vi "Move Labels in Menu.vi"(8 "error in (no error)":errorcluster caption="错误输入（无错误）", 10 "标签位置":i32[](array[numeric]), 11 "图形对象":refnum<vi>[](array[refnum])) -> (0 "error out":errorcluster caption="错误输出")   [LabVIEW 2020]
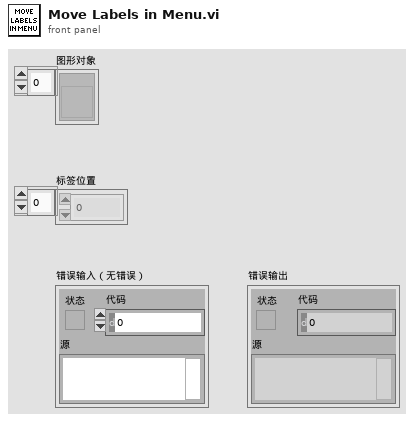
[diagram p1: front panel]
types:
  T1 = typedef "LVRectTypeDef.ctl" = cluster{"Left":i16, "Top":i16, "Right":i16, "Bottom":i16}
  T2 = cluster{"MasterRect":T1, "Label":refnum<vi>, "s? t:f":i32, refnum<vi>}
  T3 = enum32{"None", "Size to Fit", "Arrange Horizontally", "Arrange Vertically"}
  T4 = cluster{"Bounds Rect":T1, "Label":refnum<vi>, "s? t:f":i32, refnum<vi>}
  T5 = cluster{"Bounds Rect":T1, "Label":refnum<vi>, "right-top":i32, refnum<vi>}
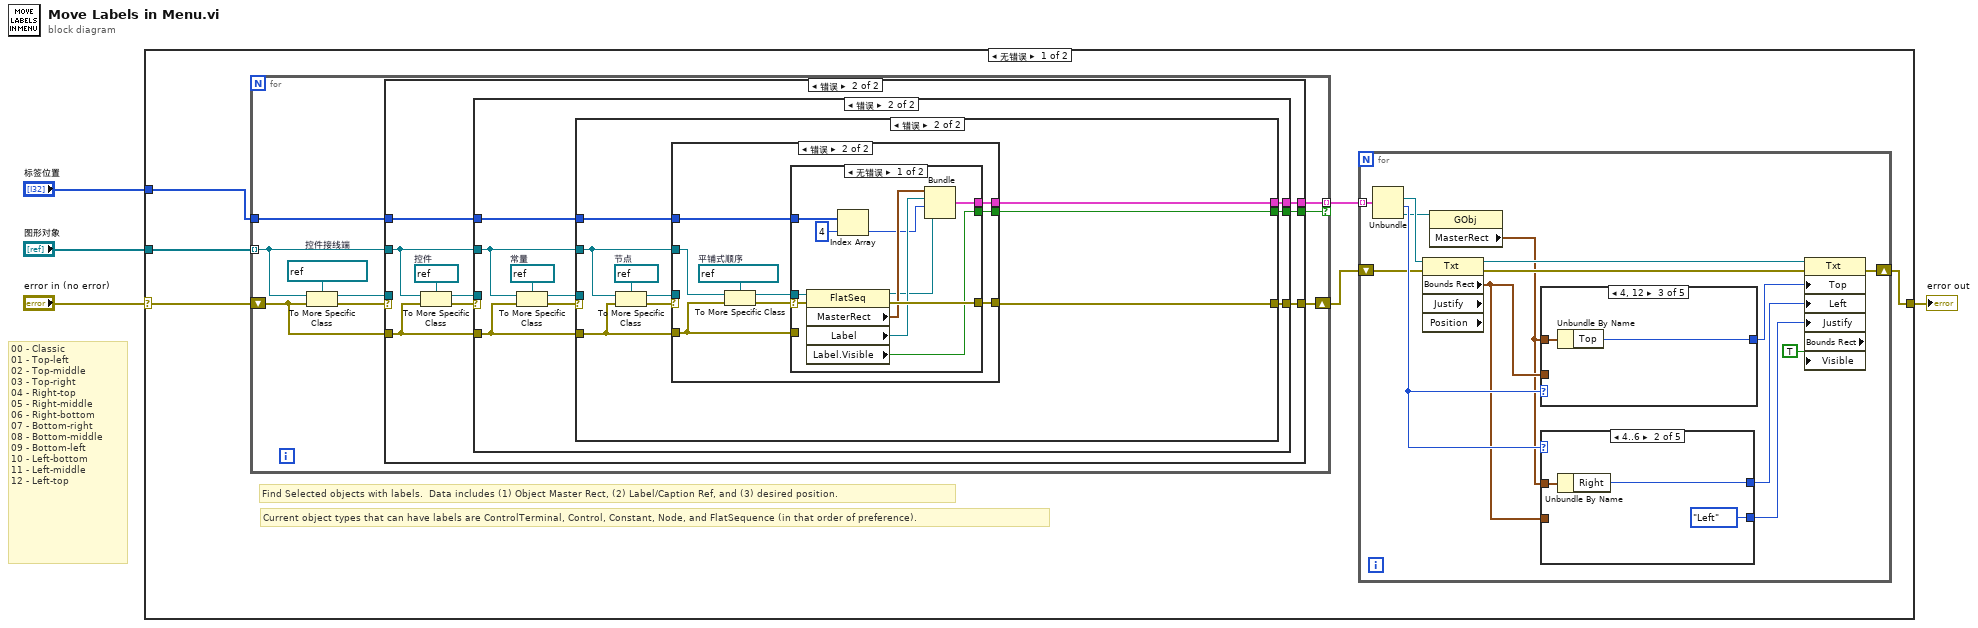
[diagram p0: block diagram]
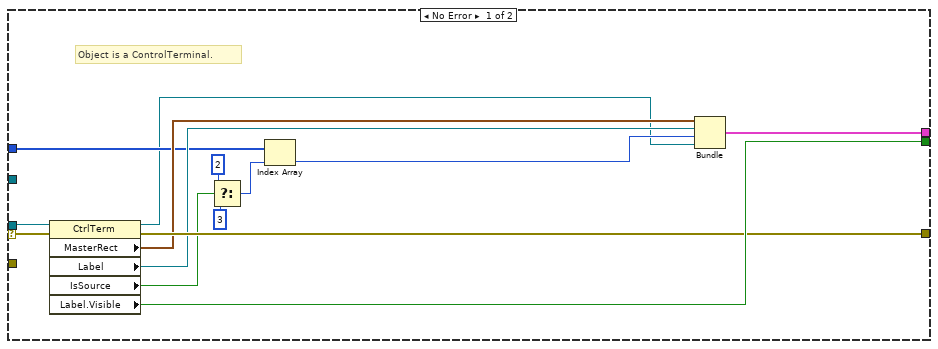
[diagram p2: hidden frame]
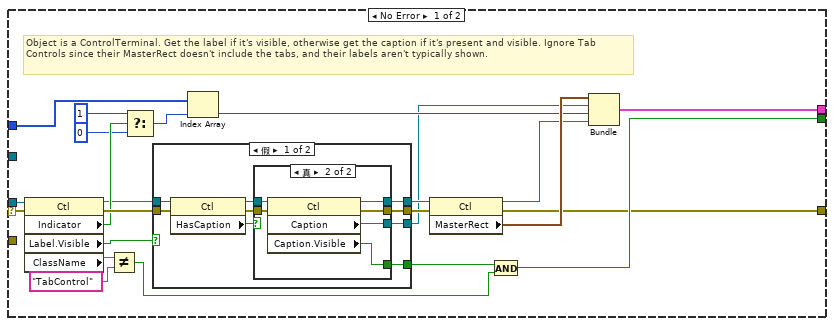
[diagram p3: hidden frame]
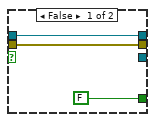
[diagram p4: hidden frame]
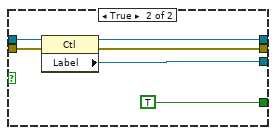
[diagram p5: hidden frame]
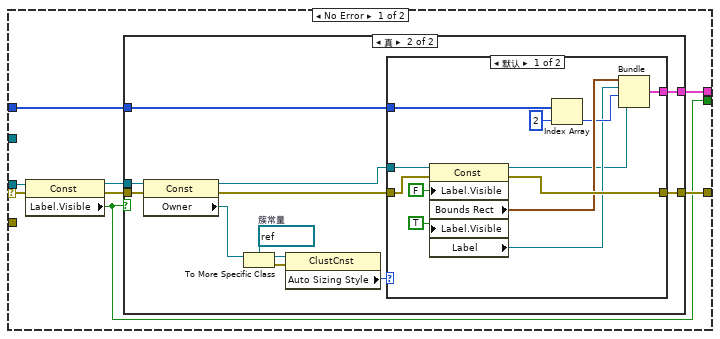
[diagram p6: hidden frame]
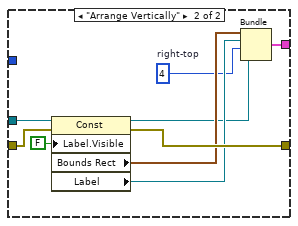
[diagram p8: hidden frame]
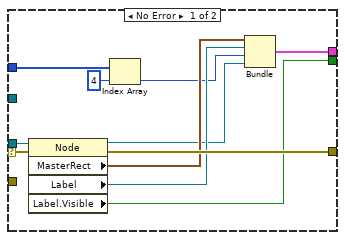
[diagram p9: hidden frame]
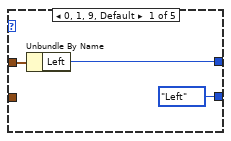
[diagram p11: hidden frame]
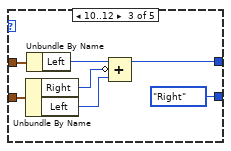
[diagram p12: hidden frame]
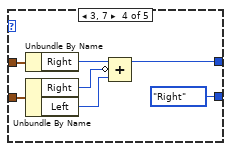
[diagram p13: hidden frame]
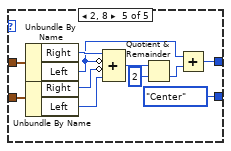
[diagram p14: hidden frame]
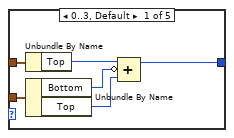
[diagram p15: hidden frame]
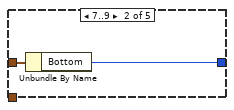
[diagram p16: hidden frame]
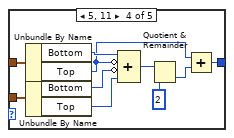
[diagram p17: hidden frame]
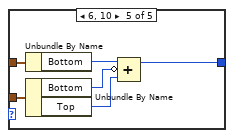
[diagram p18: hidden frame]
diagram:
  # "00 - Classic\n01 - Top-left\n02 - Top-middle\n03 - Top-right\n04 - Right-top\n05 - Right-middle\n06 - Right-bottom\n07 - Bottom-right\n08 - Bottom-middle\n09 - Bottom-left\n10 - Left-bottom\n11 - Left-middle\n12 - Left-top"
  n1 = case shown="无错误" "error in (no error)" {
    selector: "error in (no error)" -> [w8 w253]
    tunnel: [w7 w253] -> w3
    tunnel: "图形对象" -> [w6 _]
    tunnel: "标签位置" -> [w5 _]
    frame No Error {
      # "Current object types that can have labels are ControlTerminal, Control, Constant, Node, and FlatSequence (in that order of preference)."
      # "Find Selected objects with labels.  Data includes (1) Object Master Rect, (2) Label/Caption Ref, and (3) desired position."
      n2 = for {
        shift-right: [w19] -> w9
        shift-left: w8 -> [w11]
        tunnel: w6 -> [w17] mode=indexing
        tunnel: [w18] -> w10 mode=indexing if=w13
        tunnel: w5 -> [w12]
        w14 = refnum<vi> refnum  # 控件接线端
        n3 = To More Specific Class(target class=w14, reference=w17, error in=w11) -> (specific class reference=w15:refnum<vi>, error out=w16:errorcluster)
        n4 = case shown="错误" w16 {
          selector: w16 -> [w32 _]
          tunnel: [w30 w39] -> w19
          tunnel: w17 -> [_ w38]
          tunnel: [w27 w37] -> w18
          tunnel: w15 -> [w33 _]
          tunnel: [w31 w35] -> w13
          tunnel: w12 -> [w26 w36]
          tunnel: w11 -> [_ w34]
          frame No Error {
            # "Object is a ControlTerminal."
            n5 = property class="CtrlTerm"(reference=w33, error in=w32) -> (reference out=w20:refnum<vi>, error out=w30:errorcluster, "MasterRect"=w29:T1, "Label"=w28:refnum<vi>, "IsSource"=w25:bool, "Label.Visible"=w31:bool)
            n6 = Select(t=2, s=w25, f=3) -> (s? t:f=w22:i32)
            n7 = Index Array(array=w26, index=w22) -> (element=w21:i32)
            n8 = Bundle("MasterRect"=w29, "Label"=w28, "s? t:f"=w21, w20) -> (w27:T2)  [unwired: 1 in]
          }
          frame Error {
            w42 = refnum<vi> refnum  # 控件
            n9 = To More Specific Class(target class=w42, reference=w38, error in=w34) -> (specific class reference=w41:refnum<vi>, error out=w40:errorcluster)
            n10 = case shown="错误" w40 {
              selector: w40 -> [w65 _]
              tunnel: w41 -> [w61 _]
              tunnel: [w44 w94] -> w39
              tunnel: w34 -> [_ w95]
              tunnel: w38 -> [_ w93]
              tunnel: [w63 w92] -> w37
              tunnel: w36 -> [w49 w90]
              tunnel: [w46 w91] -> w35
              frame No Error {
                # "Object is a ControlTerminal. Get the label if it's visible, otherwise get the caption if it's present and visible. Ignore Tab Controls since their MasterRect doesn't include the tabs, and their labels aren't typically shown."
                n11 = property class="Ctl"(reference=w61, error in=w65) -> (reference out=w54:refnum<vi>, error out=w62:errorcluster, "Indicator"=w60:bool, "Label.Visible"=w52:bool, "ClassName"=w48:string)
                n12 = Not Equal?(x=w48, y="TabControl") -> (x != y?=w45:bool)
                n13 = Select(t=1, s=w60, f=0) -> (s? t:f=w57:i32)
                n14 = case shown="假" w52 {
                  tunnel: w62 -> [w74 w89]
                  tunnel: [w71 w86] -> w55
                  tunnel: w54 -> [w72 w88]
                  tunnel: [w69 w87] -> w53
                  tunnel: [w67 w85] -> w51
                  tunnel: [w66 TRUE] -> w50
                  frame False {
                    n15 = property class="Ctl"(reference=w72, error in=w74) -> (reference out=w70:refnum<vi>, error out=w73:errorcluster, "HasCaption"=w68:bool)
                    n16 = case shown="真" w68 {
                      tunnel: w73 -> [w76 w83]
                      tunnel: [w76 w82] -> w71
                      tunnel: w70 -> [w77 w81]
                      tunnel: [w77 w80] -> w69
                      tunnel: [_ w79] -> w67
                      tunnel: [FALSE w78] -> w66
                      frame False {
                      }
                      frame True {
                        n17 = property class="Ctl"(reference=w81, error in=w83) -> (reference out=w80:refnum<vi>, error out=w82:errorcluster, "Caption"=w79:refnum<vi>, "Caption.Visible"=w78:bool)
                      }
                    }
                  }
                  frame True {
                    n18 = property class="Ctl"(reference=w88, error in=w89) -> (reference out=w87:refnum<vi>, error out=w86:errorcluster, "Label"=w85:refnum<vi>)
                  }
                }
                n19 = Index Array(array=w49, index=w57) -> (element=w56:i32)
                n20 = property class="Ctl"(reference=w53, error in=w55) -> (reference out=w43:refnum<vi>, error out=w44:errorcluster, "MasterRect"=w64:T1)
                n21 = And(x=w50, y=w45) -> (x .and. y?=w46:bool)
                n22 = Bundle("MasterRect"=w64, "Label"=w51, "s? t:f"=w56, w43) -> (w63:T2)  [unwired: 1 in]
              }
              frame Error {
                w98 = refnum<vi> refnum  # 常量
                n23 = To More Specific Class(target class=w98, reference=w93, error in=w95) -> (specific class reference=w96:refnum<vi>, error out=w97:errorcluster)
                n24 = case shown="错误" w97 {
                  selector: w97 -> [w106 _]
                  tunnel: w95 -> [_ w145]
                  tunnel: w96 -> [w101 _]
                  tunnel: [w105 w146] -> w94
                  tunnel: w93 -> [_ w144]
                  tunnel: [w104 w143] -> w92
                  tunnel: [w99 w142] -> w91
                  tunnel: w90 -> [w103 w141]
                  frame No Error {
                    n25 = property class="Const"(reference=w101, error in=w106) -> (reference out=w100:refnum<vi>, error out=w102:errorcluster, "Label.Visible"=w99:bool)
                    n26 = case shown="真" w99 {
                      tunnel: [w107 w119] -> w105
                      tunnel: [_ w118] -> w104
                      tunnel: w103 -> [_ w117]
                      tunnel: w102 -> [w107 w116]
                      tunnel: w100 -> [_ w114]
                      frame False {
                      }
                      frame True {
                        w111 = refnum<vi> refnum  # 簇常量
                        n27 = property class="Const"(reference=w114, error in=w116) -> (reference out=w113:refnum<vi>, error out=w115:errorcluster, "Owner"=w112:refnum<vi>)
                        n28 = To More Specific Class(target class=w111, reference=w112) -> (specific class reference=w109:refnum<vi>, error out=w110:errorcluster)  [unwired: 1 in]
                        n29 = property class="ClustCnst"(reference=w109, error in=w110) -> ("Auto Sizing Style"=w108:T3)  [unwired: 2 out]
                        n30 = case shown="默认" w108 {
                          tunnel: [w131 w140] -> w119
                          tunnel: [w129 w138] -> w118
                          tunnel: w117 -> [w128 _]
                          tunnel: w115 -> [w122 w135]
                          tunnel: w113 -> [w121 w134]
                          frame Default {
                            n31 = property class="Const"(reference=w121, error in=w122, "Label.Visible"=FALSE, "Label.Visible"=TRUE) -> (reference out=w120:refnum<vi>, error out=w131:errorcluster, "Bounds Rect"=w130:T1, "Label"=w125:refnum<vi>)
                            n32 = Index Array(array=w128, index=2) -> (element=w126:i32)
                            n33 = Bundle("Bounds Rect"=w130, "Label"=w125, "s? t:f"=w126, w120) -> (w129:T4)  [unwired: 1 in]
                          }
                          frame "Arrange Vertically" {
                            w133 = 4  # right-top
                            n34 = property class="Const"(reference=w134, error in=w135, "Label.Visible"=FALSE) -> (reference out=w132:refnum<vi>, error out=w140:errorcluster, "Bounds Rect"=w139:T1, "Label"=w137:refnum<vi>)
                            n35 = Bundle("Bounds Rect"=w139, "Label"=w137, "right-top"=w133, w132) -> (w138:T5)  [unwired: 1 in]
                          }
                        }
                      }
                    }
                  }
                  frame Error {
                    w149 = refnum<vi> refnum  # 节点
                    n36 = To More Specific Class(target class=w149, reference=w144, error in=w145) -> (specific class reference=w147:refnum<vi>, error out=w148:errorcluster)
                    n37 = case shown="错误" w148 {
                      selector: w148 -> [w160 _]
                      tunnel: w147 -> [w158 _]
                      tunnel: [w159 w164] -> w146
                      tunnel: w145 -> [_ w165]
                      tunnel: w144 -> [_ w168]
                      tunnel: [w155 w163] -> w143
                      tunnel: [w154 w161] -> w142
                      tunnel: w141 -> [w153 w162]
                      frame No Error {
                        n38 = property class="Node"(reference=w158, error in=w160) -> (reference out=w150:refnum<vi>, error out=w159:errorcluster, "MasterRect"=w157:T1, "Label"=w156:refnum<vi>, "Label.Visible"=w154:bool)
                        n39 = Index Array(array=w153, index=4) -> (element=w151:i32)
                        n40 = Bundle("MasterRect"=w157, "Label"=w156, "s? t:f"=w151, w150) -> (w155:T2)  [unwired: 1 in]
                      }
                      frame Error {
                        w169 = refnum<vi> refnum  # 平铺式顺序
                        n41 = To More Specific Class(target class=w169, reference=w168, error in=w165) -> (specific class reference=w166:refnum<vi>, error out=w167:errorcluster)
                        n42 = case shown="无错误" w167 {
                          selector: w167 -> [w180 _]
                          tunnel: w166 -> [w179 _]
                          tunnel: w165 -> [_ w181]
                          tunnel: [w178 w181] -> w164
                          tunnel: [w175 _] -> w163
                          tunnel: w162 -> [w174 _]
                          tunnel: [w171 _] -> w161
                          frame No Error {
                            n43 = property class="FlatSeq"(reference=w179, error in=w180) -> (reference out=w170:refnum<vi>, error out=w178:errorcluster, "MasterRect"=w177:T1, "Label"=w176:refnum<vi>, "Label.Visible"=w171:bool)
                            n44 = Index Array(array=w174, index=4) -> (element=w172:i32)
                            n45 = Bundle("MasterRect"=w177, "Label"=w176, "s? t:f"=w172, w170) -> (w175:T2)  [unwired: 1 in]
                          }
                          frame Error {
                          }
                        }
                      }
                    }
                  }
                }
              }
            }
          }
        }
      }
      n46 = for {
        tunnel: w10 -> [w195] mode=indexing
        shift-right: [w182] -> w7
        shift-left: w9 -> [w192]
        n47 = Unbundle(w195) -> ("Label"=w193:refnum<vi>, "s? t:f"=w194:i32, w183:refnum<vi>)  [unwired: 1 out]
        n48 = property class="Txt" props=["Bounds Rect", "Justify", "Position"](reference=w193, error in=w192) -> (reference out=w191:refnum<vi>, error out=w189:errorcluster, "Bounds Rect"=w188:T1)  [unwired: 2 out]
        n49 = property class="GObj"(reference=w183) -> ("MasterRect"=w184:T1)  [unwired: 1 in, 2 out]
        n50 = case shown="4, 12" w194 {
          tunnel: w184 -> [w232 w234 w236 w246 w252]
          tunnel: w188 -> [w231 _ _ w245 w251]
          tunnel: [w227 w233 w235 w241 w247] -> w190
          frame 0..3, Default {
            n51 = Unbundle By Name(w232) -> ("Top"=w230:i16)
            n52 = Unbundle By Name(w231) -> ("Bottom"=w229:i16, "Top"=w228:i16)
            n53 = Compound Arithmetic op=ADD(w230, invert w229, w228) -> (w227:i16)
          }
          frame 7..9 {
            n54 = Unbundle By Name(w234) -> ("Bottom"=w233:i16)
          }
          frame 4, 12 {
            n55 = Unbundle By Name(w236) -> ("Top"=w235:i16)
          }
          frame 5, 11 {
            n56 = Unbundle By Name(w246) -> ("Bottom"=w240:i16, "Top"=w239:i16)
            n57 = Unbundle By Name(w245) -> ("Bottom"=w244:i16, "Top"=w243:i16)
            n58 = Compound Arithmetic op=ADD(w240, invert w239, invert w244, w243) -> (w238:i16)
            n59 = Quotient & Remainder(x=w238, y=i16 2) -> (floor(x/y)=w242:i16)  [unwired: 1 out]
            n60 = Add(x=w239, y=w242) -> (x+y=w241:i16)
          }
          frame 6, 10 {
            n61 = Unbundle By Name(w252) -> ("Bottom"=w250:i16)
            n62 = Unbundle By Name(w251) -> ("Bottom"=w249:i16, "Top"=w248:i16)
            n63 = Compound Arithmetic op=ADD(w250, invert w249, w248) -> (w247:i16)
          }
        }
        n64 = case shown="4..6" w194 {
          tunnel: w184 -> [w198 w201 w208 w215 w224]
          tunnel: w188 -> [_ _ w206 w213 w223]
          tunnel: [w197 w200 w203 w210 w220] -> w187
          tunnel: [enum16{"Left", "Center", "Right"}."Left" ("Justification") enum16{"Left", "Center", "Right"}."Left" ("Justification") enum16{"Left", "Center", "Right"}."Right" ("Justification") enum16{"Left", "Center", "Right"}."Right" ("Justification") enum16{"Left", "Center", "Right"}."Center" ("Justification")] -> w186
          frame 0, 1, 9, Default {
            n65 = Unbundle By Name(w198) -> ("Left"=w197:i16)
          }
          frame 4..6 {
            n66 = Unbundle By Name(w201) -> ("Right"=w200:i16)
          }
          frame 10..12 {
            n67 = Unbundle By Name(w206) -> ("Right"=w205:i16, "Left"=w204:i16)
            n68 = Unbundle By Name(w208) -> ("Left"=w207:i16)
            n69 = Compound Arithmetic op=ADD(w207, invert w205, w204) -> (w203:i16)
          }
          frame 3, 7 {
            n70 = Unbundle By Name(w215) -> ("Right"=w214:i16)
            n71 = Unbundle By Name(w213) -> ("Right"=w212:i16, "Left"=w211:i16)
            n72 = Compound Arithmetic op=ADD(w214, invert w212, w211) -> (w210:i16)
          }
          frame 2, 8 {
            n73 = Unbundle By Name(w224) -> ("Right"=w222:i16, "Left"=w219:i16)
            n74 = Unbundle By Name(w223) -> ("Right"=w225:i16, "Left"=w226:i16)
            n75 = Compound Arithmetic op=ADD(w222, invert w219, invert w225, w226) -> (w217:i16)
            n76 = Quotient & Remainder(x=w217, y=i16 2) -> (floor(x/y)=w221:i16)  [unwired: 1 out]
            n77 = Add(x=w219, y=w221) -> (x+y=w220:i16)
          }
        }
        n78 = property class="Txt" props=["Top", "Left", "Justify", "Bounds Rect", "Visible"](reference=w191, error in=w189, "Top"=w190, "Left"=w187, "Justify"=w186, "Visible"=TRUE) -> (error out=w182:errorcluster)  [unwired: 2 out]
      }
    }
    frame Error {
    }
  }
  "error out" <- w3
